vi "emi_Wait until MS multipl with Err.vi"(7 "millisecond multiple(0)":u32, 11 "error in (no error)":errorcluster) -> (15 "error out":errorcluster)   [LabVIEW 2011]
doc: "Same as Wait until MS multipl, but wit error in and out. \n\nRuns reentrantly, so no VI will be waiting for another with this in it.\n\nNo change in behavior due to error"
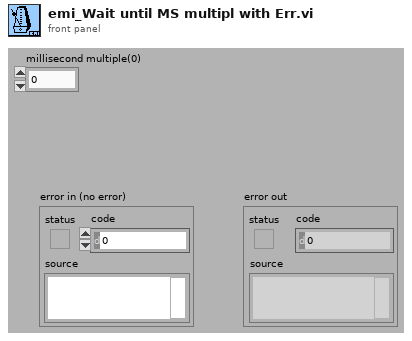
[diagram p1: front panel]
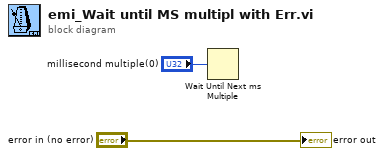
[diagram p0: block diagram]
diagram:
  n1 = Wait Until Next ms Multiple(millisecond multiple="millisecond multiple(0)") -> ()  [unwired: 1 out]
  "error out" <- "error in (no error)"
